vi "sCMOS_init.vi"(5 "error in":errorcluster {"code" format="%.0x"}, 8 "Exposure time":dbl min=1.0 max=4.0) -> (0 "error out":errorcluster {"code" format="%.0x"}, 1 "Cooler status":i32, 2 "temperature":dbl, 3 "Exposure time out":dbl, 4 "Handle out":u32)   [LabVIEW 2015]
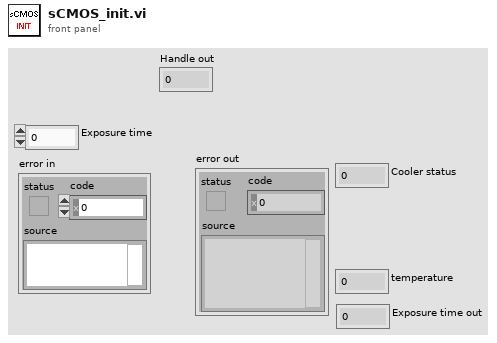
[diagram p1: front panel]
types:
  T1 = cluster{"Range":cluster{"min":dbl, "max":dbl, "step":dbl}, "default":dbl, "views":u32, "Writable":bool, "Text Values":bool, "Value Names":cluster{"Name":string, "Value":dbl}[]}
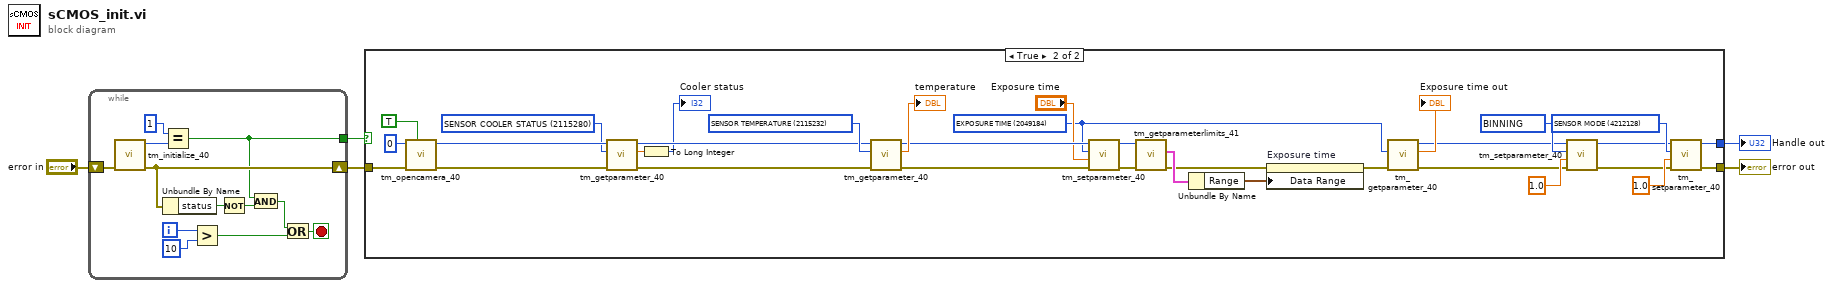
[diagram p0: block diagram]
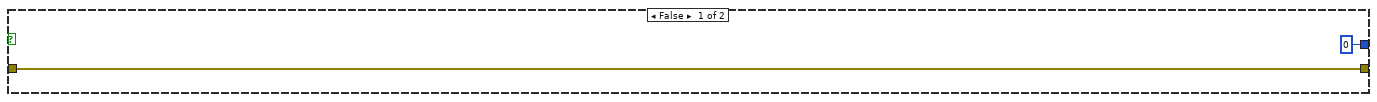
[diagram p2: hidden frame]
diagram:
  n1 = while {
    tunnel: [w9] -> w3
    shift-right: [w12] -> w4
    shift-left: "error in" -> [w17]
    i -> [w14]
    stop <- w6 stop-if-true
    n2 = call <userlib>:"tm_initialize_40.vi"("error in (no error)"=w17) -> ("error out"=w12:errorcluster, "Number Of Cameras"=w16:u32)  [unwired: 7 in, 2 out]
    n3 = Equal?(x=u32 1, y=w16) -> (x = y?=w9:bool)
    n4 = Unbundle By Name(w12) -> ("status"=w11:bool)
    n5 = Greater?(x=w14, y=10) -> (0:w7:bool)
    n6 = Not(x=w11) -> (.not. x?=w10:bool)
    n7 = And(x=w9, y=w10) -> (x .and. y?=w8:bool)
    n8 = Or(x=w8, y=w7) -> (x .or. y?=w6:bool)
  }
  n9 = case shown="True" w3 {
    tunnel: w4 -> [w19 w52]
    tunnel: [w19 w21] -> w1
    tunnel: [u32 0 ("Handle out") w20] -> w2
    frame False {
    }
    frame True {
      w24 = u32 4212128 items=["SENSOR MODE"=4212128, "READOUT SPEED"=4211872, "READOUT DIRECTION"=4211904, "TRIGGER GLOBAL EXPOSURE"=2049680, "TRIGGER DELAY"=1066480, "INTERNAL TRIGGER HANDLING"=1066496, "SYNC READOUT SYSTEM BLANK"=1066528, "SENSOR TEMPERATURE"=2115232, "SENSOR COOLER STATUS"=2115280, "EXPOSURE TIME"=2049184, "DEFECT CORRECT MODE"=4670368, "BINNING"=4215968, "INTERNAL LINE SPEED"=4226000, "INTERNAL LINE INTERVAL"=4226016, "NUMBER OF OUTPUT TRIGGER CONNECTOR"=1852320, "OUTPUT TRIGGER SOURCE[0]"=1852576, "OUTPUT TRIGGER SOURCE[1]"=1852832, "OUTPUT TRIGGER SOURCE[2]"=1853088, "OUTPUT TRIGGER POLARITY[0]"=1852592, "OUTPUT TRIGGER POLARITY[1]"=1852848, "OUTPUT TRIGGER POLARITY[2]"=1853104, "OUTPUT TRIGGER ACTIVE[0]"=1852608, "OUTPUT TRIGGER ACTIVE[1]"=1852864, "OUTPUT TRIGGER ACTIVE[2]"=1853120, "OUTPUT TRIGGER DELAY[0]"=1852624, "OUTPUT TRIGGER DELAY[1]"=1852880, "OUTPUT TRIGGER DELAY[2]"=1853136, "OUTPUT TRIGGER PERIOD[0]"=1852640, "OUTPUT TRIGGER PERIOD[1]"=1852896, "OUTPUT TRIGGER PERIOD[2]"=1853152, "OUTPUT TRIGGER KIND[0]"=1852656, "OUTPUT TRIGGER KIND[1]"=1852912, "OUTPUT TRIGGER KIND[2]"=1853168, "OUTPUT TRIGGER BASE SENSOR[0]"=1852672, "OUTPUT TRIGGER BASE SENSOR[1]"=1852928, "OUTPUT TRIGGER BASE SENSOR[2]"=1853184, "OUTPUT TRIGGER PRE HSYNC COUNT"=1852704] ("Parameter")
      w30 = u32 4215968 items=["SENSOR MODE"=4212128, "READOUT SPEED"=4211872, "READOUT DIRECTION"=4211904, "TRIGGER GLOBAL EXPOSURE"=2049680, "TRIGGER DELAY"=1066480, "INTERNAL TRIGGER HANDLING"=1066496, "SYNC READOUT SYSTEM BLANK"=1066528, "SENSOR TEMPERATURE"=2115232, "SENSOR COOLER STATUS"=2115280, "EXPOSURE TIME"=2049184, "DEFECT CORRECT MODE"=4670368, "BINNING"=4215968, "INTERNAL LINE SPEED"=4226000, "INTERNAL LINE INTERVAL"=4226016, "NUMBER OF OUTPUT TRIGGER CONNECTOR"=1852320, "OUTPUT TRIGGER SOURCE[0]"=1852576, "OUTPUT TRIGGER SOURCE[1]"=1852832, "OUTPUT TRIGGER SOURCE[2]"=1853088, "OUTPUT TRIGGER POLARITY[0]"=1852592, "OUTPUT TRIGGER POLARITY[1]"=1852848, "OUTPUT TRIGGER POLARITY[2]"=1853104, "OUTPUT TRIGGER ACTIVE[0]"=1852608, "OUTPUT TRIGGER ACTIVE[1]"=1852864, "OUTPUT TRIGGER ACTIVE[2]"=1853120, "OUTPUT TRIGGER DELAY[0]"=1852624, "OUTPUT TRIGGER DELAY[1]"=1852880, "OUTPUT TRIGGER DELAY[2]"=1853136, "OUTPUT TRIGGER PERIOD[0]"=1852640, "OUTPUT TRIGGER PERIOD[1]"=1852896, "OUTPUT TRIGGER PERIOD[2]"=1853152, "OUTPUT TRIGGER KIND[0]"=1852656, "OUTPUT TRIGGER KIND[1]"=1852912, "OUTPUT TRIGGER KIND[2]"=1853168, "OUTPUT TRIGGER BASE SENSOR[0]"=1852672, "OUTPUT TRIGGER BASE SENSOR[1]"=1852928, "OUTPUT TRIGGER BASE SENSOR[2]"=1853184, "OUTPUT TRIGGER PRE HSYNC COUNT"=1852704] ("Parameter")
      w32 = u32 2049184 items=["SENSOR MODE"=4212128, "READOUT SPEED"=4211872, "READOUT DIRECTION"=4211904, "TRIGGER GLOBAL EXPOSURE"=2049680, "TRIGGER DELAY"=1066480, "INTERNAL TRIGGER HANDLING"=1066496, "SYNC READOUT SYSTEM BLANK"=1066528, "SENSOR TEMPERATURE"=2115232, "SENSOR COOLER STATUS"=2115280, "EXPOSURE TIME"=2049184, "DEFECT CORRECT MODE"=4670368, "BINNING"=4215968, "INTERNAL LINE SPEED"=4226000, "INTERNAL LINE INTERVAL"=4226016, "NUMBER OF OUTPUT TRIGGER CONNECTOR"=1852320, "OUTPUT TRIGGER SOURCE[0]"=1852576, "OUTPUT TRIGGER SOURCE[1]"=1852832, "OUTPUT TRIGGER SOURCE[2]"=1853088, "OUTPUT TRIGGER POLARITY[0]"=1852592, "OUTPUT TRIGGER POLARITY[1]"=1852848, "OUTPUT TRIGGER POLARITY[2]"=1853104, "OUTPUT TRIGGER ACTIVE[0]"=1852608, "OUTPUT TRIGGER ACTIVE[1]"=1852864, "OUTPUT TRIGGER ACTIVE[2]"=1853120, "OUTPUT TRIGGER DELAY[0]"=1852624, "OUTPUT TRIGGER DELAY[1]"=1852880, "OUTPUT TRIGGER DELAY[2]"=1853136, "OUTPUT TRIGGER PERIOD[0]"=1852640, "OUTPUT TRIGGER PERIOD[1]"=1852896, "OUTPUT TRIGGER PERIOD[2]"=1853152, "OUTPUT TRIGGER KIND[0]"=1852656, "OUTPUT TRIGGER KIND[1]"=1852912, "OUTPUT TRIGGER KIND[2]"=1853168, "OUTPUT TRIGGER BASE SENSOR[0]"=1852672, "OUTPUT TRIGGER BASE SENSOR[1]"=1852928, "OUTPUT TRIGGER BASE SENSOR[2]"=1853184, "OUTPUT TRIGGER PRE HSYNC COUNT"=1852704] ("Parameter")
      w46 = u32 2115232 items=["SENSOR MODE"=4212128, "READOUT SPEED"=4211872, "READOUT DIRECTION"=4211904, "TRIGGER GLOBAL EXPOSURE"=2049680, "TRIGGER DELAY"=1066480, "INTERNAL TRIGGER HANDLING"=1066496, "SYNC READOUT SYSTEM BLANK"=1066528, "SENSOR TEMPERATURE"=2115232, "SENSOR COOLER STATUS"=2115280, "EXPOSURE TIME"=2049184, "DEFECT CORRECT MODE"=4670368, "BINNING"=4215968, "INTERNAL LINE SPEED"=4226000, "INTERNAL LINE INTERVAL"=4226016, "NUMBER OF OUTPUT TRIGGER CONNECTOR"=1852320, "OUTPUT TRIGGER SOURCE[0]"=1852576, "OUTPUT TRIGGER SOURCE[1]"=1852832, "OUTPUT TRIGGER SOURCE[2]"=1853088, "OUTPUT TRIGGER POLARITY[0]"=1852592, "OUTPUT TRIGGER POLARITY[1]"=1852848, "OUTPUT TRIGGER POLARITY[2]"=1853104, "OUTPUT TRIGGER ACTIVE[0]"=1852608, "OUTPUT TRIGGER ACTIVE[1]"=1852864, "OUTPUT TRIGGER ACTIVE[2]"=1853120, "OUTPUT TRIGGER DELAY[0]"=1852624, "OUTPUT TRIGGER DELAY[1]"=1852880, "OUTPUT TRIGGER DELAY[2]"=1853136, "OUTPUT TRIGGER PERIOD[0]"=1852640, "OUTPUT TRIGGER PERIOD[1]"=1852896, "OUTPUT TRIGGER PERIOD[2]"=1853152, "OUTPUT TRIGGER KIND[0]"=1852656, "OUTPUT TRIGGER KIND[1]"=1852912, "OUTPUT TRIGGER KIND[2]"=1853168, "OUTPUT TRIGGER BASE SENSOR[0]"=1852672, "OUTPUT TRIGGER BASE SENSOR[1]"=1852928, "OUTPUT TRIGGER BASE SENSOR[2]"=1853184, "OUTPUT TRIGGER PRE HSYNC COUNT"=1852704] ("Parameter")
      w48 = u32 2115280 items=["SENSOR MODE"=4212128, "READOUT SPEED"=4211872, "READOUT DIRECTION"=4211904, "TRIGGER GLOBAL EXPOSURE"=2049680, "TRIGGER DELAY"=1066480, "INTERNAL TRIGGER HANDLING"=1066496, "SYNC READOUT SYSTEM BLANK"=1066528, "SENSOR TEMPERATURE"=2115232, "SENSOR COOLER STATUS"=2115280, "EXPOSURE TIME"=2049184, "DEFECT CORRECT MODE"=4670368, "BINNING"=4215968, "INTERNAL LINE SPEED"=4226000, "INTERNAL LINE INTERVAL"=4226016, "NUMBER OF OUTPUT TRIGGER CONNECTOR"=1852320, "OUTPUT TRIGGER SOURCE[0]"=1852576, "OUTPUT TRIGGER SOURCE[1]"=1852832, "OUTPUT TRIGGER SOURCE[2]"=1853088, "OUTPUT TRIGGER POLARITY[0]"=1852592, "OUTPUT TRIGGER POLARITY[1]"=1852848, "OUTPUT TRIGGER POLARITY[2]"=1853104, "OUTPUT TRIGGER ACTIVE[0]"=1852608, "OUTPUT TRIGGER ACTIVE[1]"=1852864, "OUTPUT TRIGGER ACTIVE[2]"=1853120, "OUTPUT TRIGGER DELAY[0]"=1852624, "OUTPUT TRIGGER DELAY[1]"=1852880, "OUTPUT TRIGGER DELAY[2]"=1853136, "OUTPUT TRIGGER PERIOD[0]"=1852640, "OUTPUT TRIGGER PERIOD[1]"=1852896, "OUTPUT TRIGGER PERIOD[2]"=1853152, "OUTPUT TRIGGER KIND[0]"=1852656, "OUTPUT TRIGGER KIND[1]"=1852912, "OUTPUT TRIGGER KIND[2]"=1853168, "OUTPUT TRIGGER BASE SENSOR[0]"=1852672, "OUTPUT TRIGGER BASE SENSOR[1]"=1852928, "OUTPUT TRIGGER BASE SENSOR[2]"=1853184, "OUTPUT TRIGGER PRE HSYNC COUNT"=1852704] ("Parameter")
      n10 = call <userlib>:"tm_opencamera_40.vi"("Force Open"=TRUE, "error in (no error)"=w52, "Camera Index"=u32 0) -> ("error out"=w50:errorcluster, "Handle out"=w49:u32)  [unwired: 6 in, 1 out]
      n11 = call <userlib>:"tm_getparameter_40.vi"("error in (no error)"=w50, "Parameter"=w48, "Handle in"=w49) -> ("error out"=w44:errorcluster, "Value out"=w47:dbl, "Handle out"=w43:u32)  [unwired: 6 in]
      n12 = To Long Integer(number=w47) -> (32bit integer=→"Cooler status":i32)
      n13 = call <userlib>:"tm_getparameter_40.vi"("error in (no error)"=w44, "Parameter"=w46, "Handle in"=w43) -> ("error out"=w42:errorcluster, "Value out"=→"temperature":dbl, "Handle out"=w41:u32)  [unwired: 6 in]
      n14 = call <userlib>:"tm_setparameter_40.vi"("error in (no error)"=w42, "Value in"="Exposure time", "Parameter"=w32, "Handle in"=w41) -> ("error out"=w37:errorcluster, "Handle out"=w38:u32)  [unwired: 6 in]
      n15 = call <userlib>:"tm_getparameterlimits_41.vi"("error in (no error)"=w37, "Handle in"=w38) -> ("error out"=w36:errorcluster, "Limits"=w39:T1)  [unwired: 7 in, 1 out]
      n16 = Unbundle By Name(w39) -> ("Range"=w35:cluster{"min":dbl, "max":dbl, "step":dbl})
      n17 = property on="Exposure time" class="DigNum (strict)"(error in=w36, "Data Range"=w35) -> (error out=w34:errorcluster)  [unwired: 1 in, 1 out]
      n18 = call <userlib>:"tm_getparameter_40.vi"("error in (no error)"=w34, "Parameter"=w32) -> ("error out"=w26:errorcluster, "Value out"=→"Exposure time out":dbl, "Handle out"=w28:u32)  [unwired: 7 in]
      n19 = call <userlib>:"tm_setparameter_40.vi"("error in (no error)"=w26, "Value in"=1.0, "Parameter"=w30, "Handle in"=w28) -> ("error out"=w22:errorcluster, "Handle out"=w23:u32)  [unwired: 6 in]
      n20 = call <userlib>:"tm_setparameter_40.vi"("error in (no error)"=w22, "Value in"=1.0, "Parameter"=w24, "Handle in"=w23) -> ("error out"=w21:errorcluster, "Handle out"=w20:u32)  [unwired: 6 in]
    }
  }
  "error out" <- w1
  "Handle out" <- w2
